vi "DI Inputs -- constant.vi"() -> (2 "DI Inputs":string[](array[string])=["DI0", "DI1", "DI2", "DI3", "DI4", "DI5", "DI6", "DI7", "DI8", "DI9", "DI10", "DI11", "DI12", "DI13", "DI14", "DI15"])   [LabVIEW 2019, in "TDMS.lvlib"]
uses:
  TDMS.lvlib
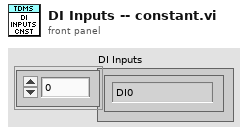
[diagram p1: front panel]
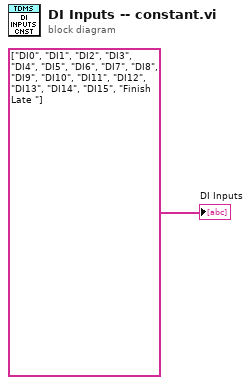
[diagram p0: block diagram]
diagram:
  "DI Inputs" <- string[] ["DI0", "DI1", "DI2", "DI3", "DI4", "DI5", "DI6", "DI7", "DI8", "DI9", "DI10", "DI11", "DI12", "DI13", "DI14", "DI15", "Finish Late "]
